vi "ReadRemoteFiles.vi"(11 "Server":path) -> ()   [LabVIEW 2020]
uses:
  ColorText/Code.xctl
panel:
  in  "Done":bool
  out "Code":string(xcontrol)="import os\n\nfor i in range(10):\n     print(i)\n"
  in  "Files":i32(listbox)
  in  "Folder":u16(ring) items=["Data"]
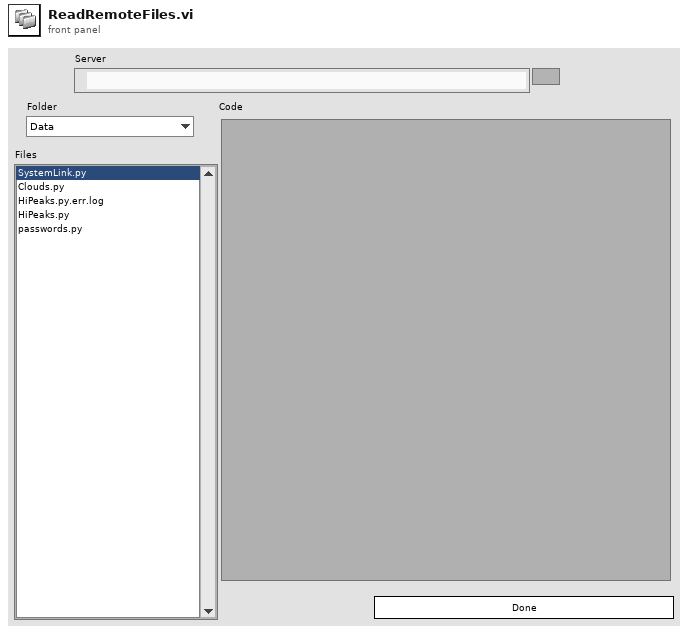
[diagram p1: front panel]
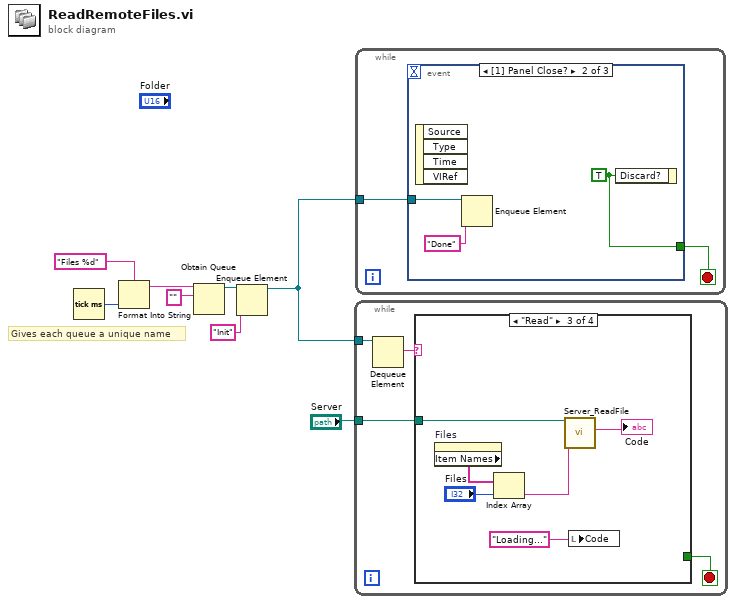
[diagram p0: block diagram]
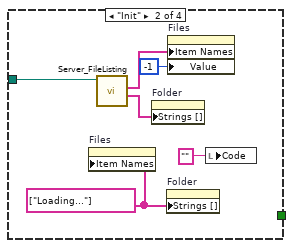
[diagram p3: hidden frame]
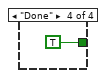
[diagram p4: hidden frame]
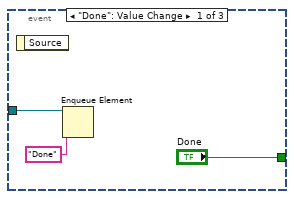
[diagram p5: hidden frame]
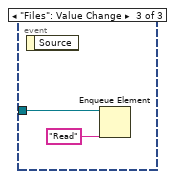
[diagram p6: hidden frame]
diagram:
  # "Gives each queue a unique name"
  n1 = Tick Count (ms)() -> (millisecond timer value=w3:u32)
  n2 = Format Into String(format string="Files %d" ("name (unnamed)"), w3) -> (resulting string=w1:string)  [unwired: 2 in, 1 out]
  n3 = Obtain Queue(name (unnamed)=w1, element data type="" ("name (unnamed)")) -> (queue out=w8:refnum<queue>)  [unwired: 3 in, 2 out]
  n4 = Enqueue Element(queue=w8, element="Init") -> (queue out=w6:refnum<queue>)  [unwired: 2 in, 2 out]
  n5 = while {
    tunnel: w6 -> [w12]
    tunnel: "Server" -> [w9]
    stop <- w10 stop-if-true
    n6 = Dequeue Element(queue=w12) -> (element=w11:string)  [unwired: 2 in, 3 out]
    n7 = case shown="\"Read\"" w11 {
      tunnel: [_ _ _ TRUE] -> w10
      tunnel: w9 -> [_ w16 w21 _]
      frame Default {
      }
      frame "Init" {
        w13 = string[] ["Loading..."] ("Item Names")
        n8 = property on="Files" class="LstBox (strict)"("Item Names"=w13) -> ()  [unwired: 2 in, 2 out]
        n9 = call "Server_FileListing.vi"("Server"=w16) -> ("Folders"=w17:string[], "Files"=w18:string[])  [unwired: 7 in, 2 out]
        n10 = property on="Folder" class="Ring (strict)"("Strings []"=w17) -> ()  [unwired: 2 in, 2 out]
        n11 = property on="Folder" class="Ring (strict)"("Strings []"=w13) -> ()  [unwired: 2 in, 2 out]
        n12 = property on="Files" class="LstBox (strict)"("Item Names"=w18, "Value"=-1 ("Files")) -> ()  [unwired: 2 in, 2 out]
        n13 = local write "Code"("") -> ()
      }
      frame "Read" {
        n14 = property on="Files" class="LstBox (strict)"() -> ("Item Names"=w24:string[])  [unwired: 2 in, 2 out]
        n15 = Index Array(array=w24, index="Files") -> (element=w22:string)
        n16 = call "Server_ReadFile.vi"("Name"=w22, "Server"=w21) -> ("Code"=→"Code":string)  [unwired: 8 in, 1 out]
        n17 = local write "Code"("Loading...") -> ()
      }
      frame "Done" {
      }
    }
  }
  n18 = while {
    tunnel: w6 -> [w26]
    stop <- w27 stop-if-true
    n19 = event shown="[1] Panel Close?" {
      selector: _ -> [_ _ _]
      dyn-events: _ -> [_ _ _]
      timeout: _ -> [_ _ _]
      tunnel: ["Done" w31 _] -> w27
      tunnel: w26 -> [w28 w32 w34]
      event "Done": Value Change {
        n20 = event-data() -> ()  [unwired: 1 in, 1 out]
        n21 = Enqueue Element(queue=w28, element="Done") -> ()  [unwired: 2 in, 3 out]
      }
      event Panel Close? {
        w31 = TRUE ("Discard?")
        n22 = event-data() -> ()  [unwired: 1 in, 4 out]
        n23 = Enqueue Element(queue=w32, element="Done") -> ()  [unwired: 2 in, 3 out]
        n24 = event-data("Discard?"=w31) -> ()  [unwired: 1 in, 1 out]
      }
      event "Files": Value Change {
        n25 = event-data() -> ()  [unwired: 1 in, 1 out]
        n26 = Enqueue Element(queue=w34, element="Read") -> ()  [unwired: 2 in, 3 out]
      }
    }
  }
